vi "TX_IMD3(DEBUG) .vi"() -> ()   [LabVIEW 2015]
uses:
  <instrlib>/Rohde&Schwarz Spectrum Analyzer/Rohde&Schwarz Spectrum Analyzer.lvlib
panel:
  in  "TWO TONE STEP(MHz)":u32=5
  in  "O_R&S Spec1 2":refnum<visa-resource-name>
  in  "O_R&S Spec1":refnum<visa-resource-name>="GPIB0::22::INSTR"
  out "B通道发射带":cluster{"X":dbl[], "Amplitude":dbl[]}(graph)
  out "A通道发射带":cluster{"X":dbl[], "Amplitude":dbl[]}(graph)
  out "B_peak":dbl[](array[numeric])
  out "B_pos":dbl[](array[numeric])
  out "B_next_pos":dbl[](array[numeric])
  out "B_peak_next":dbl[](array[numeric])
  out "Array 6":cluster{"X":dbl[], "Amplitude":dbl[]}[](array[cluster])
  out "A_peak":dbl[](array[numeric])
  out "A_pos":dbl[](array[numeric])
  out "A_next_pos":dbl[](array[numeric])
  out "A_peak_next":dbl[](array[numeric])
  out "Array":cluster{"X":dbl[], "Amplitude":dbl[]}[](array[cluster])
  in  "OK":bool
  in  "stop":bool
  out "Bx":dbl[](array[numeric]) caption="X" format="%^.3e"
  out "By":dbl[](array[numeric]) caption="Amplitude" format="%^.3e"
  out "B_pos":dbl caption="Marker Position" format="%^.3e"
  out "B_peak":dbl caption="Marker Amplitude" format="%^.3e"
  out "A_peak":dbl caption="Marker Amplitude" format="%^.3e"
  out "A_pos":dbl caption="Marker Position" format="%^.3e"
  out "Ay":dbl[](array[numeric]) caption="Amplitude" format="%^.3e"
  out "Ax":dbl[](array[numeric]) caption="X" format="%^.3e"
  in  "VISA resource name 2":refnum<visa-resource-name>="COM3"
  out "Freq_Tab":u32[](array[numeric])
  in  "Value":u32=3 caption="Point Num"
  in  "cnt/setp":enum16{"SETP", "COUNT"}(ring)=enum."COUNT"
  in  "freq_max(Mhz)":u32=2123
  in  "freq_min(Mhz)":u32=2018
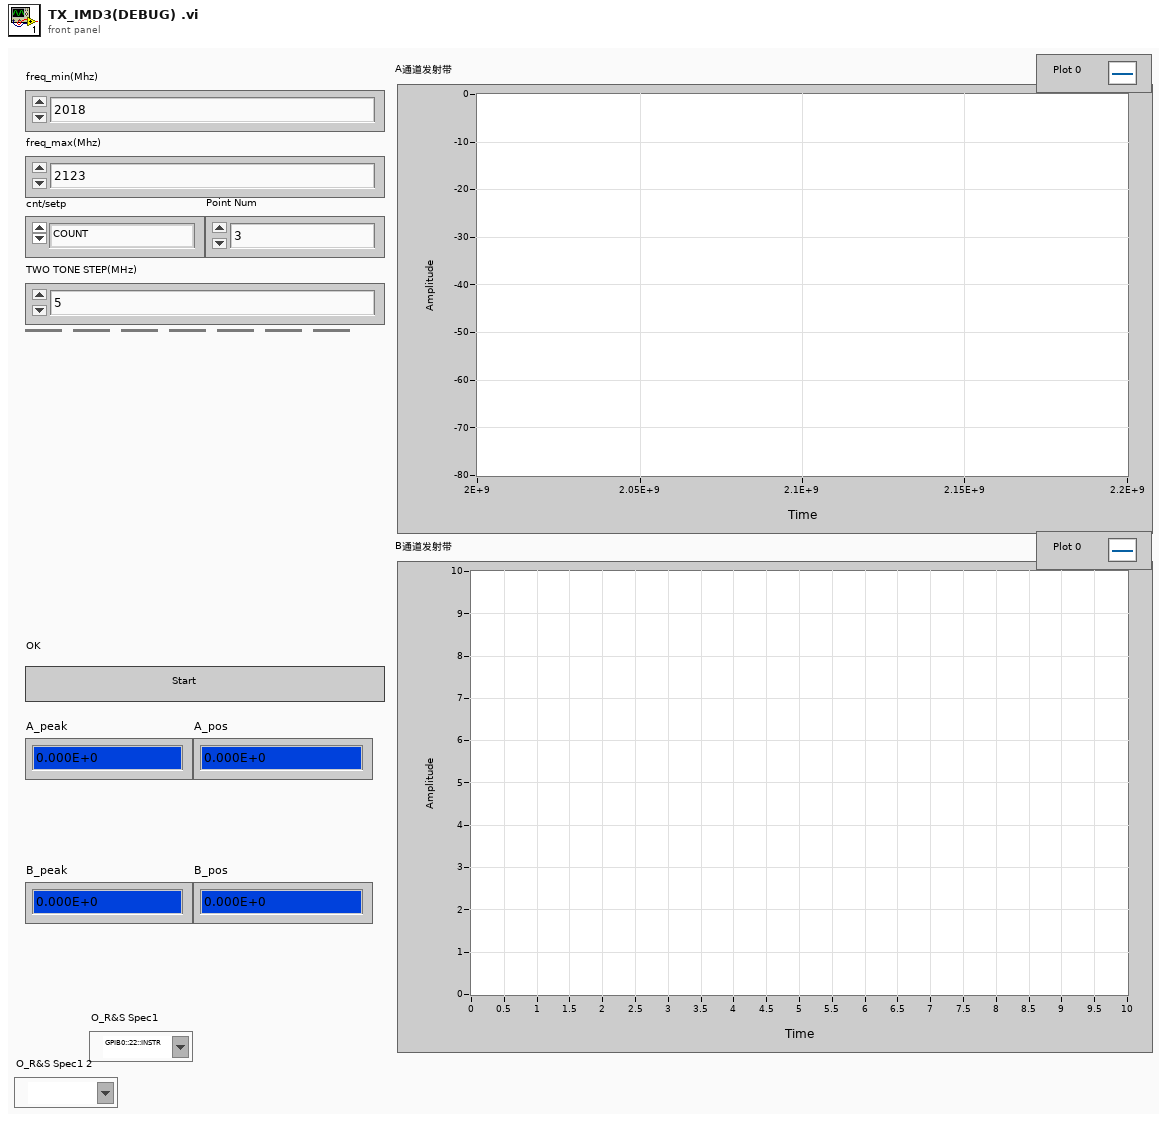
[diagram p1: front panel]
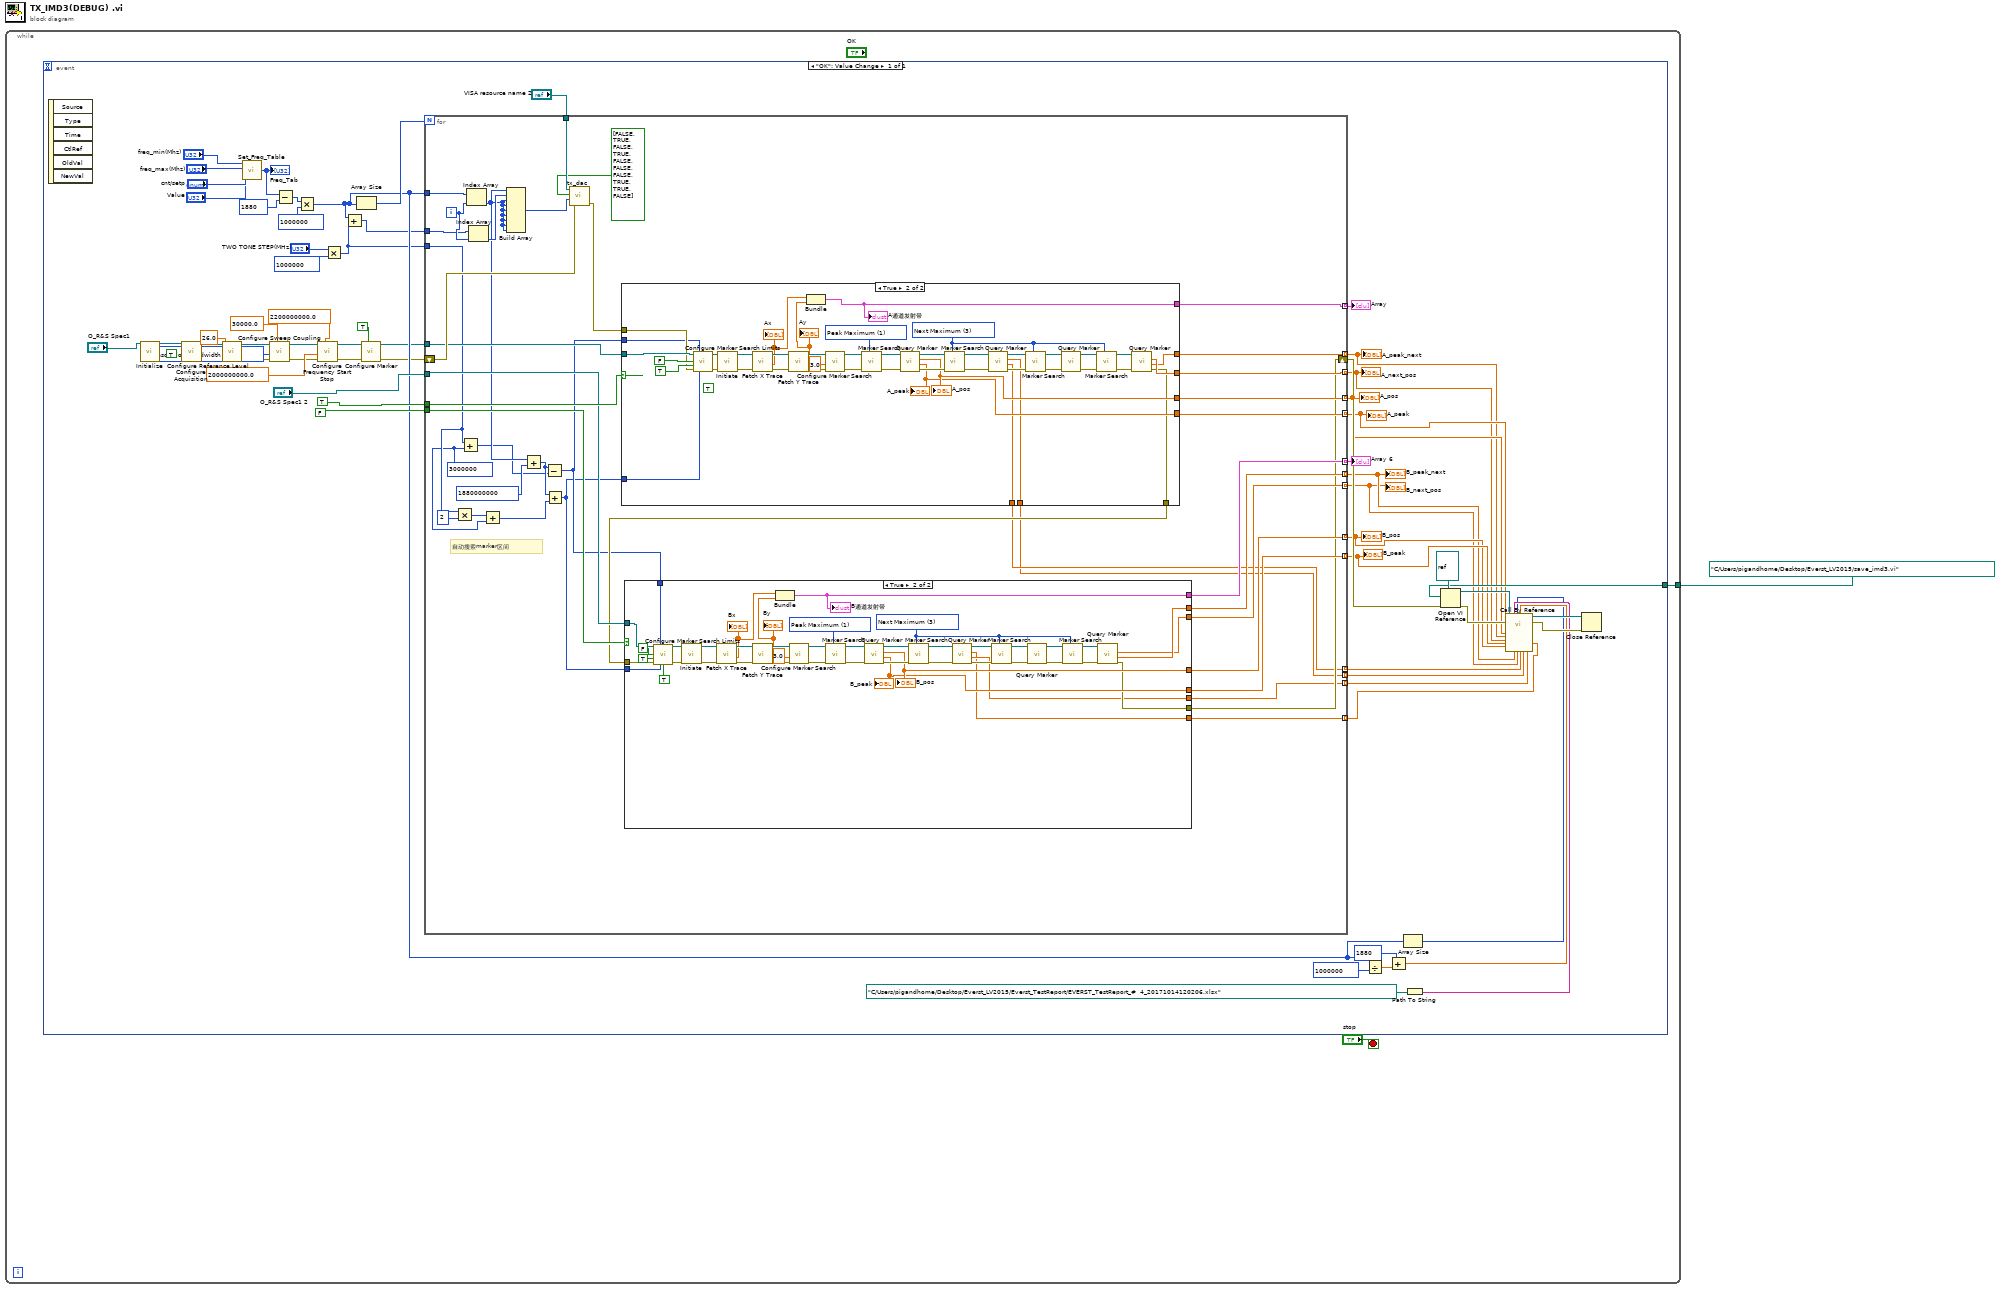
[diagram p0: block diagram]
diagram:
  n1 = while {
    tunnel: path "C:/Users/pigandhome/Desktop/Everst_LV2015/save_imd3.vi" ("vi path") -> [w2]
    stop <- "stop" stop-if-true
    n2 = event shown="[0] \"OK\": Value Change" {
      selector: _ -> [_]
      dyn-events: _ -> [_]
      timeout: _ -> [_]
      tunnel: w2 -> [w51]
      event "OK": Value Change {
        w10 = 0 items=["Resolution Bandwidth", "Video Bandwidth", "Sweep Time"] ("Sweep Coupling (Resolution Bandwidth)")
        n3 = event-data() -> ()  [unwired: 1 in, 6 out]
        n4 = call <instrlib>:"Initialize.vi"("VISA resource name"="O_R&S Spec1") -> ("VISA resource name out"=w26:refnum<visa-resource-name>, "error out"=w27:errorcluster)  [unwired: 13 in]
        n5 = call <instrlib>:"Configure Acquisition.vi"("error in (no error)"=w27, "Sweep Mode Continuous (F: Off)"=TRUE, "VISA resource name"=w26) -> ("error out"=w25:errorcluster, "VISA resource name out"=w24:refnum<visa-resource-name>)  [unwired: 7 in]
        n6 = call <instrlib>:"Configure Reference Level.vi"("error in (no error)"=w25, "Reference Level (-20.0)"=26.0, "VISA resource name"=w24) -> ("error out"=w14:errorcluster, "VISA resource name out"=w13:refnum<visa-resource-name>)  [unwired: 7 in]
        n7 = call "Set_Freq_Table.vi"("Value"="Value", "cnt/setp"="cnt/setp", "freq_max(Mhz)"="freq_max(Mhz)", "freq_min(Mhz)"="freq_min(Mhz)") -> ("Freq_Tab"=w65:u32[])  [unwired: 2 in]
        "Freq_Tab" <- w65
        n8 = call <instrlib>:"Configure Sweep Coupling.vi"("Coupling Value (0.0)"=30000.0, "error in (no error)"=w14, "Sweep Coupling (Resolution Bandwidth)"=w10, "VISA resource name"=w13) -> ("error out"=w12:errorcluster, "VISA resource name out"=w11:refnum<visa-resource-name>)  [unwired: 6 in]
        n9 = Subtract(x=w65, y=1880) -> (x-y=w63:u32[])
        n10 = Multiply(x=w63, y=1000000) -> (x*y=w32:u32[])
        n11 = call <instrlib>:"Configure Frequency Start Stop.vi"("Stop Frequency (0.0)"=2200000000.0 ("Start Frequency (0.0)"), "error in (no error)"=w12, "Start Frequency (0.0)"=2000000000.0, "VISA resource name"=w11) -> ("error out"=w23:errorcluster, "VISA resource name out"=w22:refnum<visa-resource-name>)  [unwired: 6 in]
        n12 = Multiply(x="TWO TONE STEP(MHz)", y=u32 1000000) -> (x*y=w8:u32)
        n13 = Add(x=w32, y=w8) -> (x+y=w31:u32[])
        n14 = Array Size(array=w32) -> (size(s)=w61:i32)
        n15 = call <instrlib>:"Configure Marker.vi"("Marker State (F: Off)"=TRUE, "error in (no error)"=w23, "VISA resource name"=w22) -> ("error out"=w21:errorcluster, "VISA resource name out"=w20:refnum<visa-resource-name>)  [unwired: 7 in]
        n16 = for {
          N: w61 -> [_]
          tunnel: w32 -> [w109]
          tunnel: "VISA resource name 2" -> [w108]
          tunnel: w20 -> [w93]
          tunnel: "O_R&S Spec1 2" -> [w91]
          tunnel: TRUE ("spec1_state") -> [w94]
          tunnel: FALSE ("spec1_state") -> [w92]
          shift-right: [w85] -> w52
          shift-left: w21 -> [w105]
          tunnel: [w104] -> w39 mode=indexing
          tunnel: [w103] -> w38 mode=indexing
          tunnel: [w102] -> w40 mode=indexing
          tunnel: [w101] -> w41 mode=indexing
          tunnel: [w100] -> w34 mode=indexing
          tunnel: [w99] -> w35 mode=indexing
          tunnel: [w98] -> w36 mode=indexing
          tunnel: [w97] -> w37 mode=indexing
          tunnel: [w96] -> w59 mode=indexing
          tunnel: [w95] -> w58 mode=indexing
          tunnel: w31 -> [w88]
          tunnel: w8 -> [w78]
          tunnel: [w73] -> w7 mode=indexing
          tunnel: [w72] -> w6 mode=indexing
          tunnel: [w71] -> w5 mode=indexing
          tunnel: [w70] -> w4 mode=indexing
          i -> [w89]
          w75 = u32 3000000 ("y")
          # "自动搜索marker区间"
          n17 = Multiply(x=w78, y=u32 2) -> (x*y=w76:u32)
          n18 = Add(x=w78, y=w75) -> (x+y=w79:u32)
          n19 = Index Array(array=w109, index=w89) -> (element=w84:u32)
          n20 = Index Array(array=w88, index=w89) -> (element=w87:u32)
          n21 = Add(x=w76, y=w75) -> (x+y=w74:u32)
          n22 = Build Array(w84, w87, w84, w84, w84, w84, w84, w84, w84) -> (w107:u32[])
          n23 = Add(x=w84, y=u32 1880000000) -> (x+y=w82:u32)
          n24 = Subtract(x=w82, y=w79) -> (x-y=w81:u32)
          n25 = Add(x=w82, y=w74) -> (x+y=w80:u32)
          n26 = call "tx_dac.vi"("error in (no error)"=w105, "fin"=w107, "开关"=bool[] [FALSE, TRUE, FALSE, TRUE, FALSE, FALSE, FALSE, TRUE, TRUE, FALSE], "VISA resource name 2"=w108) -> ("error out"=w106:errorcluster)  [unwired: 2 in]
          n27 = case shown="True" w94 {
            tunnel: w93 -> [_ w173]
            tunnel: w106 -> [w155 w172]
            tunnel: [_ w161] -> w104
            tunnel: [_ w162] -> w103
            tunnel: [_ w182] -> w102
            tunnel: [_ w181] -> w101
            tunnel: [_ w178] -> w96
            tunnel: [w155 w160] -> w86
            tunnel: w81 -> [_ w158]
            tunnel: w80 -> [_ w159]
            tunnel: [_ w157] -> w73
            tunnel: [_ w156] -> w72
            frame False {
            }
            frame True {
              (unwired) TRUE ("Search Limits Zoom (F: Off)")
              w163 = 3 items=["Peak Maximum"=1, "Peak Minimum"=2, "Next Maximum"=3, "Left Maximum"=4, "Right Maximum"=5, "Next Minimum"=6, "Left Minimum"=7, "Right Minimum"=8] ("Marker Search (Peak Maximum)")
              w183 = 1 items=["Peak Maximum"=1, "Peak Minimum"=2, "Next Maximum"=3, "Left Maximum"=4, "Right Maximum"=5, "Next Minimum"=6, "Left Minimum"=7, "Right Minimum"=8] ("Marker Search (Peak Maximum)")
              n28 = call <instrlib>:"Configure Marker Search Limits.vi"("VISA resource name"=w173, "Search Limit Left (0.0)"=w158, "Threshold State (T: On)"=FALSE, "Search Limits (F: Off)"=TRUE, "error in (no error)"=w172, "Search Limit Right (0.0)"=w159) -> ("VISA resource name out"=w176:refnum<visa-resource-name>, "error out"=w177:errorcluster)  [unwired: 8 in]
              n29 = call <instrlib>:"Initiate.vi"("error in (no error)"=w177, "VISA resource name"=w176) -> ("error out"=w198:errorcluster, "VISA resource name out"=w197:refnum<visa-resource-name>)  [unwired: 8 in]
              n30 = call <instrlib>:"Fetch X Trace.vi"("error in (no error)"=w198, "VISA resource name"=w197) -> ("error out"=w196:errorcluster, "X"=w180:dbl[], "VISA resource name out"=w195:refnum<visa-resource-name>)  [unwired: 7 in]
              "Ax" <- w180
              n31 = call <instrlib>:"Fetch Y Trace.vi"("error in (no error)"=w196, "VISA resource name"=w195) -> ("error out"=w194:errorcluster, "Amplitude"=w179:dbl[], "VISA resource name out"=w193:refnum<visa-resource-name>)  [unwired: 7 in]
              "Ay" <- w179
              n32 = Bundle("X"=w180, "Amplitude"=w179) -> (w178:cluster{"X":dbl[], "Amplitude":dbl[]})  [unwired: 1 in]
              "A通道发射带" <- w178
              n33 = call <instrlib>:"Configure Marker Search.vi"("error in (no error)"=w194, "Peak Excursion (6.0)"=3.0, "VISA resource name"=w193) -> ("error out"=w192:errorcluster, "VISA resource name out"=w191:refnum<visa-resource-name>)  [unwired: 7 in]
              n34 = call <instrlib>:"Marker Search.vi"("Marker Search (Peak Maximum)"=w183, "error in (no error)"=w192, "VISA resource name"=w191) -> ("error out"=w190:errorcluster, "VISA resource name out"=w189:refnum<visa-resource-name>)  [unwired: 7 in]
              n35 = call <instrlib>:"Query Marker.vi"("error in (no error)"=w190, "VISA resource name"=w189) -> ("error out"=w188:errorcluster, "Marker Amplitude"=w181:dbl, "Marker Position"=w182:dbl, "VISA resource name out"=w187:refnum<visa-resource-name>)  [unwired: 6 in]
              "A_pos" <- w182
              "A_peak" <- w181
              n36 = call <instrlib>:"Marker Search.vi"("Marker Search (Peak Maximum)"=w163, "error in (no error)"=w188, "VISA resource name"=w187) -> ("error out"=w186:errorcluster, "VISA resource name out"=w185:refnum<visa-resource-name>)  [unwired: 7 in]
              n37 = call <instrlib>:"Query Marker.vi"("error in (no error)"=w186, "VISA resource name"=w185) -> ("error out"=w171:errorcluster, "Marker Amplitude"=w157:dbl, "Marker Position"=w156:dbl, "VISA resource name out"=w170:refnum<visa-resource-name>)  [unwired: 6 in]
              n38 = call <instrlib>:"Marker Search.vi"("Marker Search (Peak Maximum)"=w163, "error in (no error)"=w171, "VISA resource name"=w170) -> ("error out"=w169:errorcluster, "VISA resource name out"=w168:refnum<visa-resource-name>)  [unwired: 7 in]
              n39 = call <instrlib>:"Query Marker.vi"("error in (no error)"=w169, "VISA resource name"=w168) -> ("error out"=w167:errorcluster, "VISA resource name out"=w166:refnum<visa-resource-name>)  [unwired: 6 in, 2 out]
              n40 = call <instrlib>:"Marker Search.vi"("Marker Search (Peak Maximum)"=w163, "error in (no error)"=w167, "VISA resource name"=w166) -> ("error out"=w165:errorcluster, "VISA resource name out"=w164:refnum<visa-resource-name>)  [unwired: 7 in]
              n41 = call <instrlib>:"Query Marker.vi"("error in (no error)"=w165, "VISA resource name"=w164) -> ("error out"=w160:errorcluster, "Marker Amplitude"=w161:dbl, "Marker Position"=w162:dbl)  [unwired: 6 in, 1 out]
            }
          }
          n42 = case shown="True" w92 {
            tunnel: w91 -> [_ w120]
            tunnel: w86 -> [w110 w121]
            tunnel: [_ w124] -> w100
            tunnel: [_ w125] -> w99
            tunnel: [_ w138] -> w98
            tunnel: [_ w137] -> w97
            tunnel: [_ w134] -> w95
            tunnel: [w110 w118] -> w85
            tunnel: w81 -> [_ w117]
            tunnel: w80 -> [_ w116]
            tunnel: [_ w112] -> w71
            tunnel: [_ w111] -> w70
            frame False {
            }
            frame True {
              w123 = 3 items=["Peak Maximum"=1, "Peak Minimum"=2, "Next Maximum"=3, "Left Maximum"=4, "Right Maximum"=5, "Next Minimum"=6, "Left Minimum"=7, "Right Minimum"=8] ("Marker Search (Peak Maximum)")
              w154 = 1 items=["Peak Maximum"=1, "Peak Minimum"=2, "Next Maximum"=3, "Left Maximum"=4, "Right Maximum"=5, "Next Minimum"=6, "Left Minimum"=7, "Right Minimum"=8] ("Marker Search (Peak Maximum)")
              n43 = call <instrlib>:"Configure Marker Search Limits.vi"("VISA resource name"=w120, "Search Limit Left (0.0)"=w117, "Threshold State (T: On)"=FALSE, "Search Limits (F: Off)"=TRUE, "error in (no error)"=w121, "Search Limit Right (0.0)"=w116, "Search Limits Zoom (F: Off)"=TRUE) -> ("VISA resource name out"=w119:refnum<visa-resource-name>, "error out"=w122:errorcluster)  [unwired: 7 in]
              n44 = call <instrlib>:"Initiate.vi"("error in (no error)"=w122, "VISA resource name"=w119) -> ("error out"=w139:errorcluster, "VISA resource name out"=w140:refnum<visa-resource-name>)  [unwired: 8 in]
              n45 = call <instrlib>:"Fetch X Trace.vi"("error in (no error)"=w139, "VISA resource name"=w140) -> ("error out"=w141:errorcluster, "X"=w136:dbl[], "VISA resource name out"=w142:refnum<visa-resource-name>)  [unwired: 7 in]
              "Bx" <- w136
              n46 = call <instrlib>:"Fetch Y Trace.vi"("error in (no error)"=w141, "VISA resource name"=w142) -> ("error out"=w143:errorcluster, "Amplitude"=w135:dbl[], "VISA resource name out"=w144:refnum<visa-resource-name>)  [unwired: 7 in]
              "By" <- w135
              n47 = Bundle("X"=w136, "Amplitude"=w135) -> (w134:cluster{"X":dbl[], "Amplitude":dbl[]})  [unwired: 1 in]
              "B通道发射带" <- w134
              n48 = call <instrlib>:"Configure Marker Search.vi"("error in (no error)"=w143, "Peak Excursion (6.0)"=3.0, "VISA resource name"=w144) -> ("error out"=w145:errorcluster, "VISA resource name out"=w146:refnum<visa-resource-name>)  [unwired: 7 in]
              n49 = call <instrlib>:"Marker Search.vi"("Marker Search (Peak Maximum)"=w154, "error in (no error)"=w145, "VISA resource name"=w146) -> ("error out"=w147:errorcluster, "VISA resource name out"=w148:refnum<visa-resource-name>)  [unwired: 7 in]
              n50 = call <instrlib>:"Query Marker.vi"("error in (no error)"=w147, "VISA resource name"=w148) -> ("error out"=w149:errorcluster, "Marker Amplitude"=w137:dbl, "Marker Position"=w138:dbl, "VISA resource name out"=w150:refnum<visa-resource-name>)  [unwired: 6 in]
              "B_pos" <- w138
              "B_peak" <- w137
              n51 = call <instrlib>:"Marker Search.vi"("Marker Search (Peak Maximum)"=w123, "error in (no error)"=w149, "VISA resource name"=w150) -> ("error out"=w151:errorcluster, "VISA resource name out"=w152:refnum<visa-resource-name>)  [unwired: 7 in]
              n52 = call <instrlib>:"Query Marker.vi"("error in (no error)"=w151, "VISA resource name"=w152) -> ("error out"=w133:errorcluster, "Marker Amplitude"=w112:dbl, "Marker Position"=w111:dbl, "VISA resource name out"=w132:refnum<visa-resource-name>)  [unwired: 6 in]
              n53 = call <instrlib>:"Marker Search.vi"("Marker Search (Peak Maximum)"=w123, "error in (no error)"=w133, "VISA resource name"=w132) -> ("error out"=w131:errorcluster, "VISA resource name out"=w130:refnum<visa-resource-name>)  [unwired: 7 in]
              n54 = call <instrlib>:"Query Marker.vi"("error in (no error)"=w131, "VISA resource name"=w130) -> ("error out"=w129:errorcluster, "VISA resource name out"=w128:refnum<visa-resource-name>)  [unwired: 6 in, 2 out]
              n55 = call <instrlib>:"Marker Search.vi"("Marker Search (Peak Maximum)"=w123, "error in (no error)"=w129, "VISA resource name"=w128) -> ("error out"=w127:errorcluster, "VISA resource name out"=w126:refnum<visa-resource-name>)  [unwired: 7 in]
              n56 = call <instrlib>:"Query Marker.vi"("error in (no error)"=w127, "VISA resource name"=w126) -> ("error out"=w118:errorcluster, "Marker Amplitude"=w125:dbl, "Marker Position"=w124:dbl)  [unwired: 6 in, 1 out]
            }
          }
        }
        "Array" <- w59
        "A_peak_next" <- w39
        "A_next_pos" <- w38
        "A_pos" <- w40
        "A_peak" <- w41
        "Array 6" <- w58
        "B_peak_next" <- w35
        "B_next_pos" <- w34
        "B_pos" <- w36
        "B_peak" <- w37
        n57 = Divide(x=w32, y=u32 1000000) -> (x/y=w44:dbl[])
        n58 = Add(x=u32 1880, y=w44) -> (x+y=w42:dbl[])
        n59 = Array Size(array=w32) -> (size(s)=w33:i32)
        n60 = Path To String(path=path "C:/Users/pigandhome/Desktop/Everst_LV2015/Everst_TestReport/EVERST_TestReport_#  4_20171014120206.xlsx") -> (string=w50:string)
        n61 = Open VI Reference(type specifier VI Refnum (for type only)=refnum<vi> refnum, vi path=w51, error in (no error)=w52) -> (vi reference=w57:refnum<vi>, error out=w56:errorcluster)  [unwired: 3 in]
        n62 = call-by-ref "?"(reference=w57, error in=w56, "Apeak"=w41, "Apeakpos"=w40, "Apeaknext"=w39, "Anextpos"=w38, "Bpeak"=w37, "Bpeakpos"=w36, "PATH"=w50, "Bpeaknext"=w35, "Tabsize"=w33, "Bnextpos"=w34, "FreqTab"=w42, "RApeak"=w7, "RApos"=w6, "RBpos"=w4, "RBpeak"=w5) -> (reference out=w53:refnum<vi>, error out=w54:errorcluster)  [unwired: 5 in]
        n63 = Close Reference(reference=w53, error in (no error)=w54) -> ()  [unwired: 1 out]
      }
    }
  }
